vi "Analyse Board.vi"(8 "error in (no error)":errorcluster, 10 "GameBoard":u8[][](array[numeric]), 11 "CS++GoBangServer in":refnum<class "CS++GoBangServer.lvclass">) -> (0 "error out":errorcluster, 3 "CS++GoBangServer out":refnum<class "CS++GoBangServer.lvclass">)   [LabVIEW 2013, in "GoBang.lvlib" / "CS++GoBangServer.lvclass"]
uses:
  CS++GoBangServer.lvclass
  Core/Classes/CS++ProcessVariables/ProcessVariable/PV.lvclass
  typdefs/GameState.ctl
  CS++GoBangServer.lvclass/CS++GoBangServer.ctl
  Core/Classes/CS++ProcessVariables/ProcessVariable/PV.lvclass/PV.ctl
  Core/Classes/CS++ProcessVariables/PVConnection/PVConnection.lvclass
  Core/Classes/CS++ProcessVariables/ProcessVariable/Write Data.vi
  Core/Classes/CS++ProcessVariables/ProcessVariable/Write Timestamp.vi
  Core/Classes/CS++ProcessVariables/ProcessVariable/Write Quality.vi
  Core/Classes/CS++ProcessVariables/ProcessVariable/Write status.vi
  GoBang.lvlib
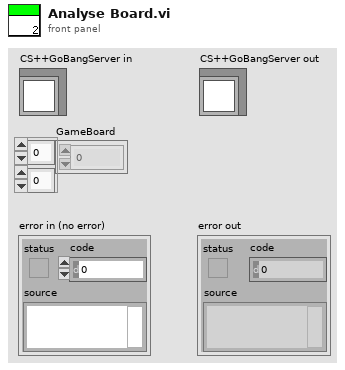
[diagram p1: front panel]
types:
  T1 = typedef "GoBang.lvlib/GameState.ctl" = enum16{"Waiting for opponent", "White to move", "Black to move", "Game over, white won", "Game over, black won"}
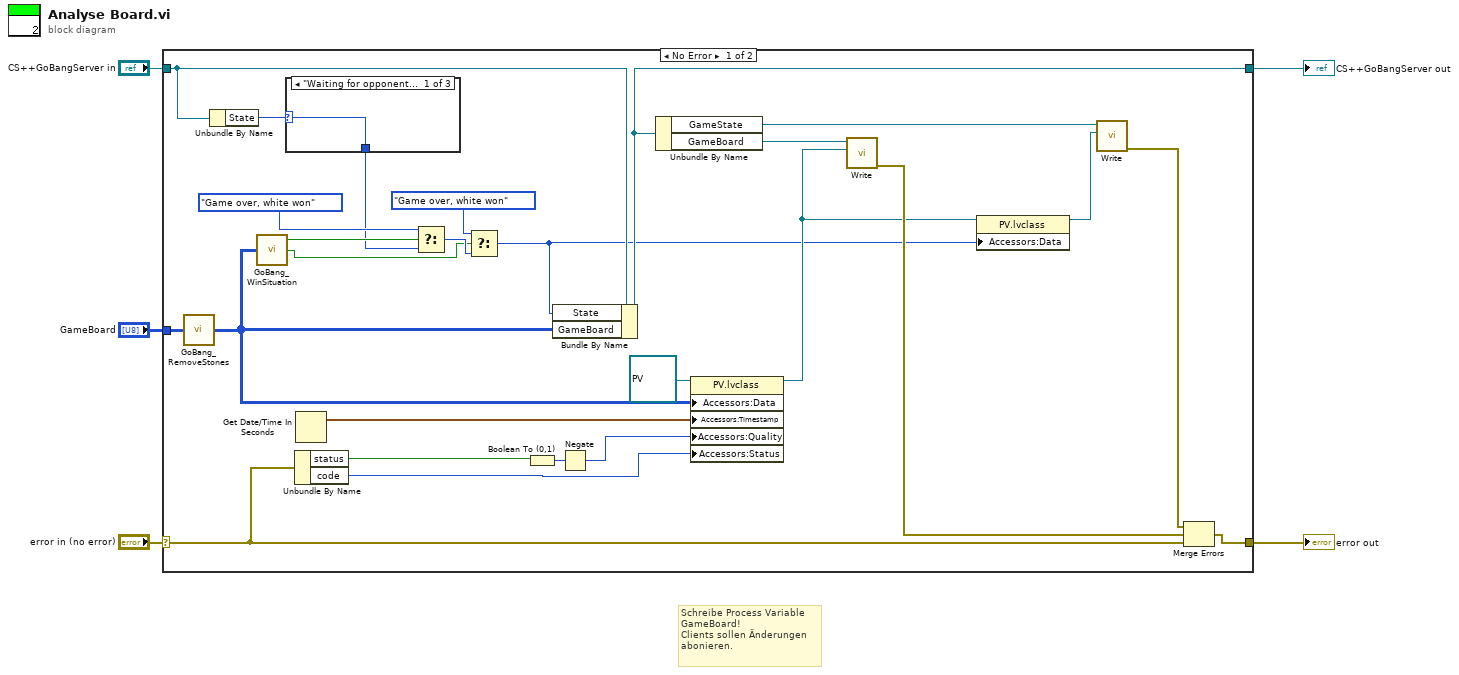
[diagram p0: block diagram]
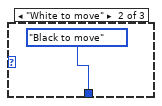
[diagram p2: hidden frame]
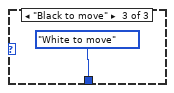
[diagram p3: hidden frame]
diagram:
  # "Schreibe Process Variable \nGameBoard!\nClients sollen Änderungen\nabonieren."
  n1 = case shown="No Error" "error in (no error)" {
    selector: "error in (no error)" -> [w25 w36]
    tunnel: [w20 w36] -> w4
    tunnel: [w30 w35] -> w2
    tunnel: "CS++GoBangServer in" -> [w12 w35]
    tunnel: "GameBoard" -> [w31 _]
    frame No Error {
      n2 = call "GoBang_RemoveStones.vi"("GameBoard in"=w31) -> ("GameBoard out"=w21:u8[][])
      n3 = Unbundle By Name(w12) -> ("State"=w8:T1)
      n4 = call "GoBang_WinSituation.vi"("GameBoard"=w21) -> ("White won"=w14:bool, "Black won"=w10:bool)  [unwired: 1 out]
      n5 = case shown="\"Waiting for opponent\", Default" w8 {
        selector: w8 -> [w32 _ _]
        tunnel: [w32 GameState."Black to move" ("State") GameState."White to move" ("State")] -> w7
        frame "Waiting for opponent", Default {
        }
        frame "White to move" {
        }
        frame "Black to move" {
        }
      }
      n6 = Unbundle By Name(w25) -> ("status"=w26:bool, "code"=w23:i32)
      n7 = Get Date/Time In Seconds() -> (seconds since 1Jan1904=w22:timestamp)
      n8 = Select(t=GameState."Game over, white won" ("State"), s=w14, f=w7) -> (s? t:f=w11:T1)
      n9 = Select(t=GameState."Game over, white won" ("State"), s=w10, f=w11) -> (s? t:f=w6:T1)
      n10 = Boolean To (0,1)(Boolean=w26) -> (0, 1=w27:i16)
      n11 = Bundle By Name(cluster=w12, "State"=w6, "GameBoard"=w21) -> (w30:refnum<class "CS++GoBangServer.lvclass">)
      n12 = Negate(x=w27) -> (-x=w24:i16)
      n13 = Unbundle By Name(w30) -> ("GameState"=w18:refnum<class "PVConnection.lvclass">, "GameBoard"=w29:refnum<class "PVConnection.lvclass">)
      n14 = property class="PV.lvclass"(reference=refnum<class "PV.lvclass"> refnum ("CS++ProcessVariables.lvlib:PV.lvclass"), "Accessors:Data"=w21, "Accessors:Timestamp"=w22, "Accessors:Quality"=w24, "Accessors:Status"=w23) -> (reference out=w17:refnum<class "PV.lvclass">)  [unwired: 1 in, 1 out]
      n15 = call-dynamic "Write.vi"("PV"=w17, "PVConnection in"=w29) -> ("error out"=w19:errorcluster)  [unwired: 8 in, 1 out]
      n16 = property class="PV.lvclass"(reference=w17, "Accessors:Data"=w6) -> (reference out=w16:refnum<class "PV.lvclass">)  [unwired: 1 in, 1 out]
      n17 = call-dynamic "Write.vi"("PV"=w16, "PVConnection in"=w18) -> ("error out"=w15:errorcluster)  [unwired: 8 in, 1 out]
      n18 = Merge Errors(w15, w19, w25) -> (w20:errorcluster)
    }
    frame Error {
    }
  }
  "error out" <- w4
  "CS++GoBangServer out" <- w2
